vi "UTL_PopulateGlobalsWithCtrlNumber.vi"(8 "error in (no error)":errorcluster) -> (0 "error out":errorcluster)   [LabVIEW 2019]
uses:
  Variable global de carga.vi
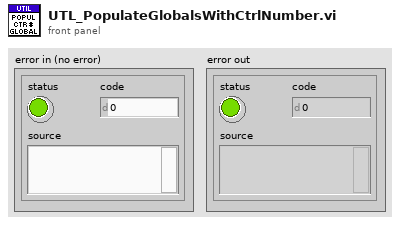
[diagram p1: front panel]
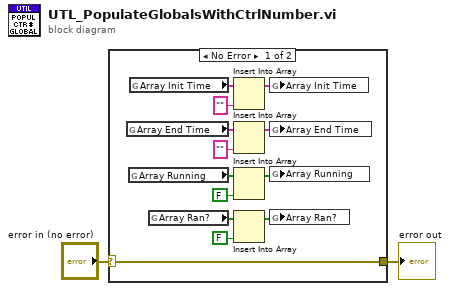
[diagram p0: block diagram]
diagram:
  n1 = case shown="No Error" "error in (no error)" {
    selector: "error in (no error)" -> [w15 w16]
    tunnel: [w15 w16] -> w1
    frame No Error {
      n2 = global read "Variable global de carga.vi" "Array End Time"() -> (w11:string[])
      n3 = global read "Variable global de carga.vi" "Array Running"() -> (w10:bool[])
      n4 = global read "Variable global de carga.vi" "Array Init Time"() -> (w14:string[])
      n5 = global read "Variable global de carga.vi" "Array Ran?"() -> (w7:bool[])
      n6 = Insert Into Array(array=w14, new element="" ("new element/subarray")) -> (w13:string[])  [unwired: 1 in]
      n7 = Insert Into Array(array=w11, new element="" ("new element/subarray")) -> (w12:string[])  [unwired: 1 in]
      n8 = Insert Into Array(array=w10, new element=FALSE) -> (w9:bool[])  [unwired: 1 in]
      n9 = Insert Into Array(array=w7, new element=FALSE) -> (w8:bool[])  [unwired: 1 in]
      n10 = global write "Variable global de carga.vi" "Array Init Time"(w13) -> ()
      n11 = global write "Variable global de carga.vi" "Array End Time"(w12) -> ()
      n12 = global write "Variable global de carga.vi" "Array Running"(w9) -> ()
      n13 = global write "Variable global de carga.vi" "Array Ran?"(w8) -> ()
    }
    frame Error {
    }
  }
  "error out" <- w1
